vi "Spectrometer_File_Naming.vi"(9 "Description":string, 10 "Sample MetaData Cluster":T1={"Sample Volume (uL)"=18.0, "Sample Mass (ug)"=0.45, "Sample Conc(mg/mL)"=0.025, "Sample Temperature (C)"=23.0, "Batch Num"=999.0, "Batch Name"="Test", "Solute"="Test", "Solvent"="Water", "Sample Description"="Test"}, 11 "Ring":u16(ring)=3 items=["Spec.", "Mag.", "In Out Spec", "SRM", "", ""]) -> (3 "Output Name":string="SRM_Test_")   [LabVIEW 2021]
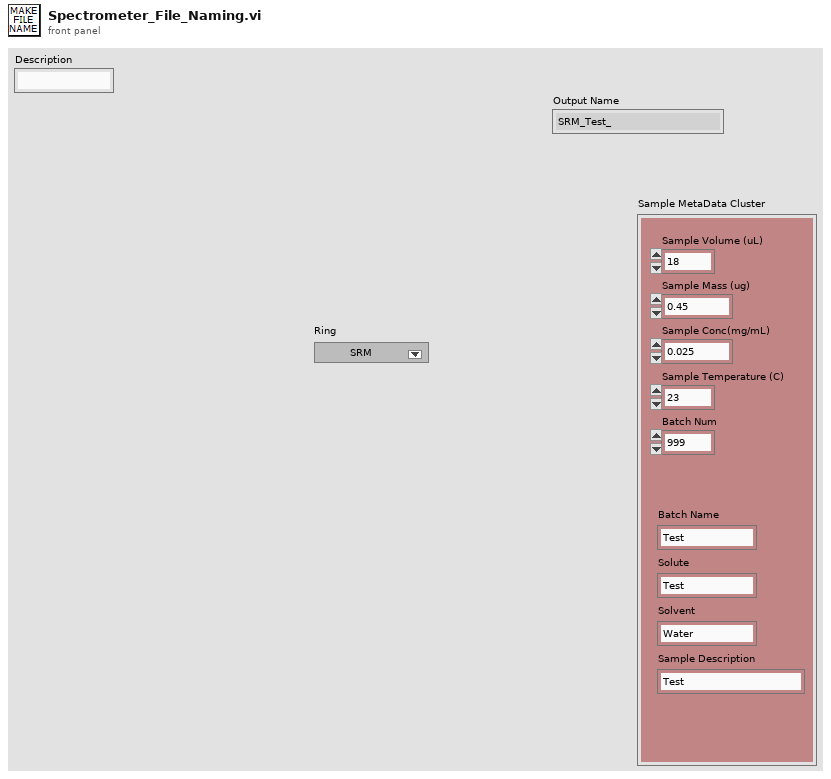
[diagram p1: front panel]
types:
  T1 = cluster{"Sample Volume (uL)":dbl, "Sample Mass (ug)":dbl, "Sample Conc(mg/mL)":dbl, "Sample Temperature (C)":dbl, "Batch Num":dbl, "Batch Name":string, "Solute":string, "Solvent":string, "Sample Description":string}
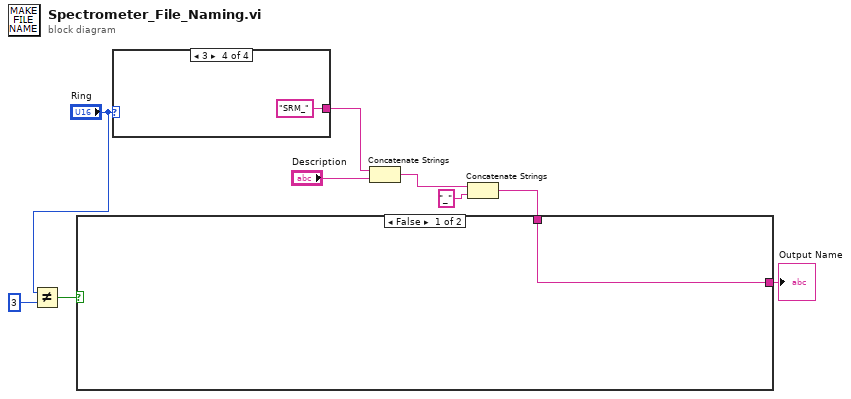
[diagram p0: block diagram]
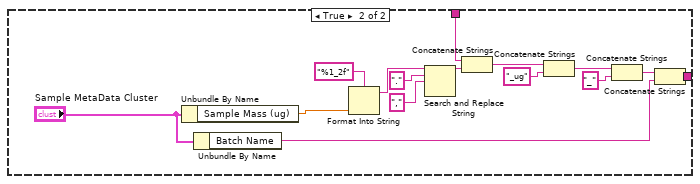
[diagram p2: hidden frame]
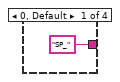
[diagram p3: hidden frame]
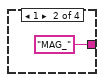
[diagram p4: hidden frame]
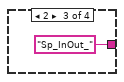
[diagram p5: hidden frame]
diagram:
  n1 = Not Equal?(x="Ring", y=u16 3) -> (x != y?=w1:bool)
  n2 = case shown="3" "Ring" {
    tunnel: ["SP_" ("string") "MAG_" ("string") "Sp_InOut_" ("string") "SRM_" ("string")] -> w7
    frame 0, Default {
    }
    frame 1 {
    }
    frame 2 {
    }
    frame 3 {
    }
  }
  n3 = Concatenate Strings(w7, "Description") -> (w4:string)
  n4 = Concatenate Strings(w4, "_" ("string")) -> (w5:string)
  n5 = case shown="False" w1 {
    tunnel: [w14 w21] -> w9
    tunnel: w5 -> [w14 w15]
    frame False {
    }
    frame True {
      n6 = Unbundle By Name("Sample MetaData Cluster") -> ("Sample Mass (ug)"=w29:dbl)
      n7 = Unbundle By Name("Sample MetaData Cluster") -> ("Batch Name"=w20:string)
      n8 = Format Into String(format string="%1_2f", w29) -> (resulting string=w25:string)  [unwired: 2 in, 1 out]
      n9 = Search and Replace String(input string=w25, search string=".", replace string="," ("replace string (\"\")")) -> (result string=w22:string)  [unwired: 5 in, 3 out]
      n10 = Concatenate Strings(w15, w22) -> (w27:string)
      n11 = Concatenate Strings(w27, "_ug" ("string")) -> (w18:string)
      n12 = Concatenate Strings(w18, "_" ("string")) -> (w16:string)
      n13 = Concatenate Strings(w16, w20) -> (w21:string)
    }
  }
  "Output Name" <- w9
